vi "SmartSEM Remote API grid voltage.vi"(7 "Iterations":u32=3, 8 "error in":errorcluster, 9 "Grid voltage":sgl, 10 "Det Type":string, 11 "ActiveX Container":refnum<k7>(container)) -> (0 "error out":errorcluster, 3 "reference out":refnum<k7>)   [LabVIEW 2018]
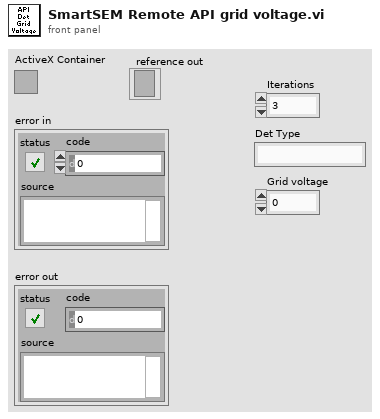
[diagram p1: front panel]
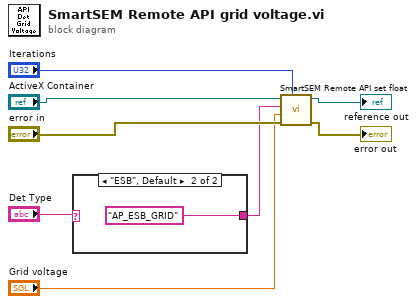
[diagram p0: block diagram]
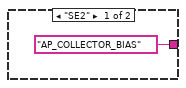
[diagram p2: hidden frame]
diagram:
  n1 = case shown="\"ESB\", Default" "Det Type" {
    tunnel: ["AP_COLLECTOR_BIAS" ("lpszCommand") "AP_ESB_GRID" ("lpszCommand")] -> w4
    frame "SE2" {
    }
    frame "ESB", Default {
    }
  }
  n2 = call "SmartSEM Remote API set float.vi"("Iterations"="Iterations", "error in"="error in", "vValue"="Grid voltage", "lpszParam"=w4, "ActiveX Container"="ActiveX Container") -> ("error out"=→"error out":errorcluster, "reference out"=→"reference out":refnum<k7>)  [unwired: 5 in]
